vi "y1y2 副本.vi"(6 "二值化输入":u8[][](array[numeric]), 9 "Image Pixels (U8)输入":u8[][](array[numeric])) -> (0 "out right point 2":cluster{i32, i32}[](array[cluster]), 1 "right":cluster{i32, i32}[](graph), 2 "out left point":cluster{i32, i32}[](array[cluster]), 3 "left":cluster{i32, i32}[](graph), 4 "四个角点":i32[][](array[numeric]))   [LabVIEW 2014]
panel:
  out "x2max":cluster{i32, i32}
  out "x2min":cluster{i32, i32}
  out "x1min":cluster{i32, i32}
  out "x1max":cluster{i32, i32}
  # "x"
  # "1"
  # "2"
  # "y"
  # "x"
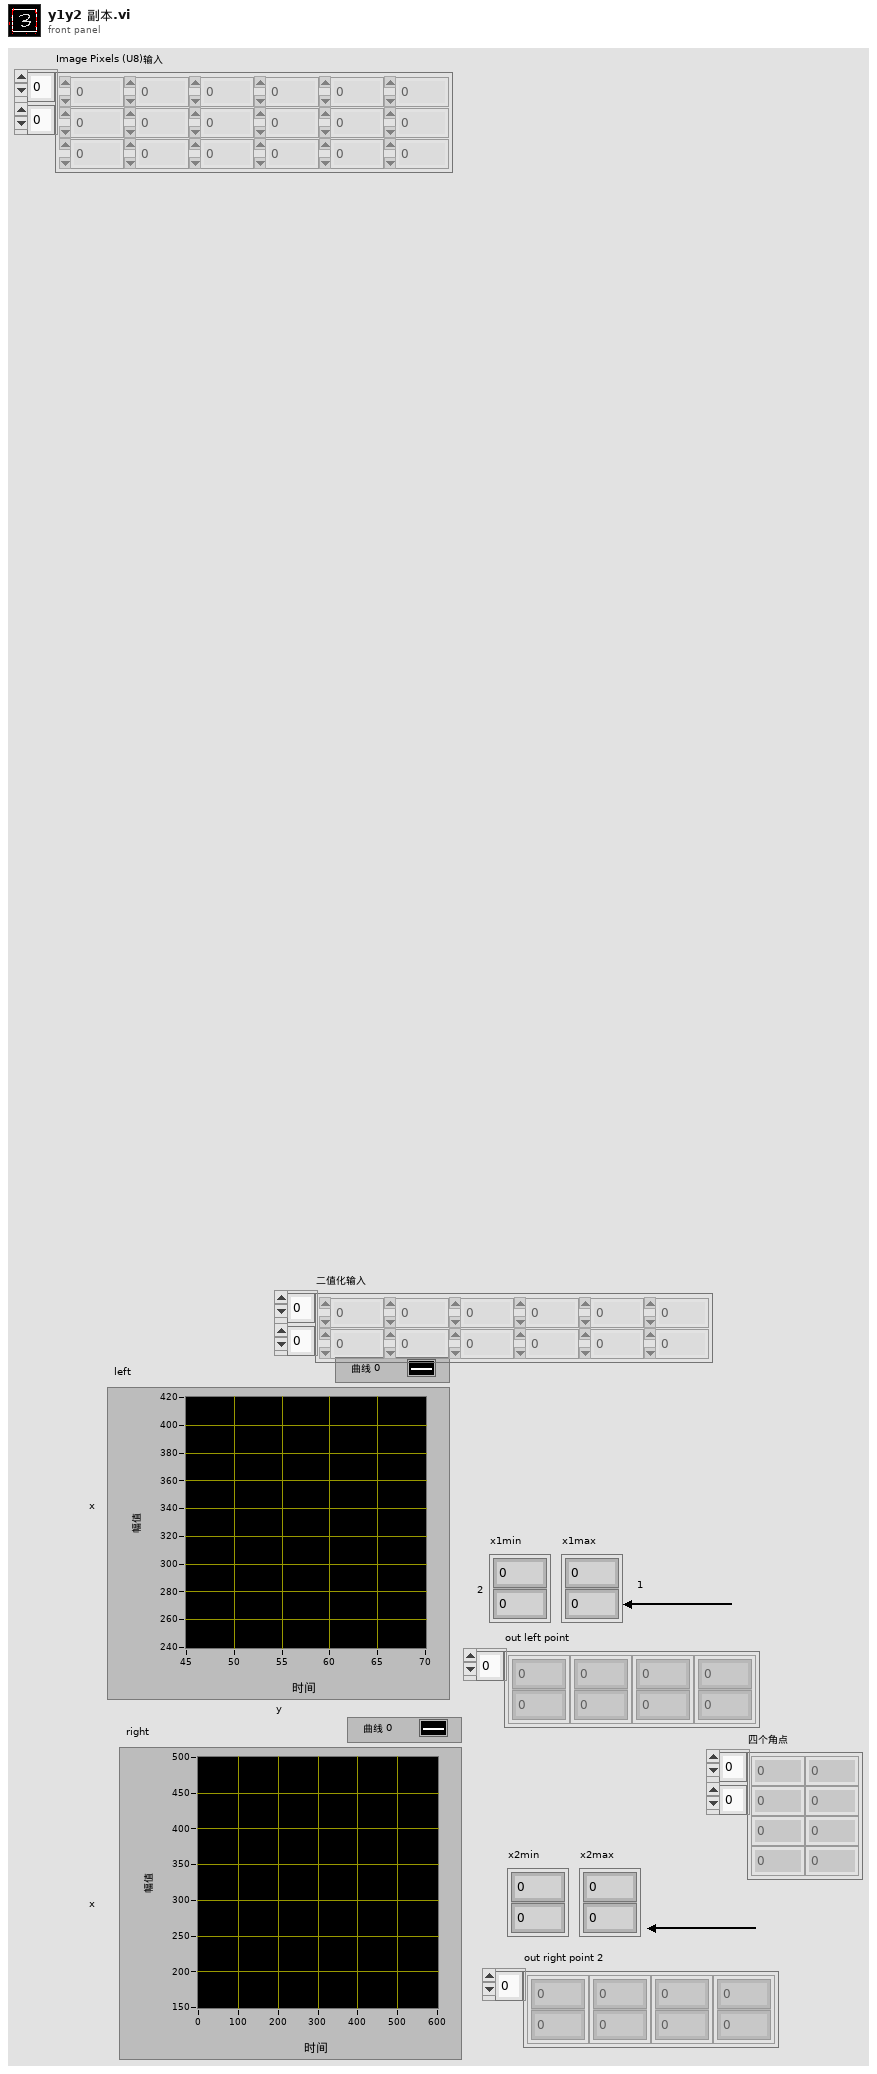
[diagram p1: front panel]
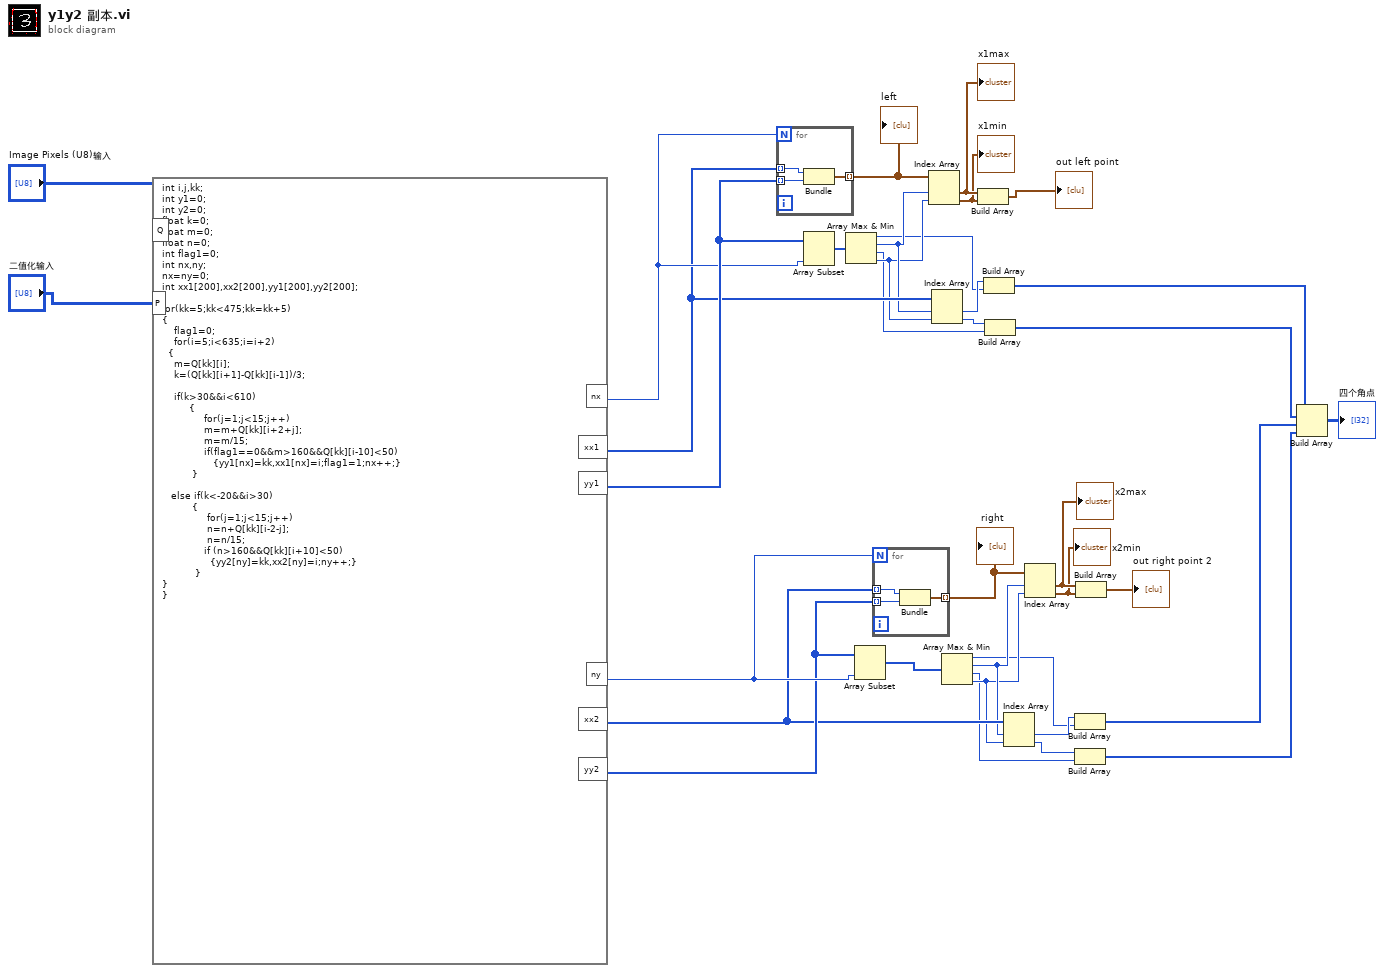
[diagram p0: block diagram]
diagram:
  n1 = formula code="int i,j,kk;\nint y1=0;\nint y2=0;\nfloat k=0;\nfloat m=0;\nfloat n=0;\nint flag1=0;\nint nx,ny;\nnx=ny=0;\nint xx1[200],xx2[200],yy1[200],yy2[200];\n\nfor(kk=5;kk<475;kk=kk+5)\n{\n    flag1=0;\n    for(i=5;i<635;i=i+2)\n  {\n    m=Q[kk][i];\n    k=(Q[kk][i+1]-Q[kk][i-1])/3;\n\n    if(k>30&&i<610)\n         {   \n              for(j=1;j<15;j++)\n              m=m+Q[kk][i+2+j];\n              m=m/15;\n              if(flag1==0&&m>160&&Q[kk][i-10]<50)\n                 {yy1[nx]=kk,xx1[nx]=i;flag1=1;nx++;}\n          }\n\n   else if(k<-20&&i>30)\n          {                   \n               for(j=1;j<15;j++)\n               n=n+Q[kk][i-2-j];\n               n=n/15;\n              if (n>160&&Q[kk][i+10]<50)\n                {yy2[ny]=kk,xx2[ny]=i;ny++;}\n           }\n}\n}"("Q"="Image Pixels (U8)输入", "P"="二值化输入") -> ("xx1"=w20:i32[], "yy1"=w34:i32[], "nx"=w33:i32, "xx2"=w10:i32[], "yy2"=w30:i32[], "ny"=w31:i32)
  n2 = for {
    N: w33 -> [_]
    tunnel: w20 -> [w38] mode=indexing
    tunnel: w34 -> [w37] mode=indexing
    tunnel: [w36] -> w35 mode=indexing
    n3 = Bundle(w38, w37) -> (w36:cluster{i32, i32})  [unwired: 1 in]
  }
  "left" <- w35
  n4 = Array Subset(array=w34, length=w33) -> (w23:i32[])  [unwired: 1 in]
  n5 = Array Max & Min(array=w23) -> (max value=w16:i32, max index (indices)=w19:i32, min value=w14:i32, min index (indices)=w18:i32)
  n6 = Array Subset(array=w30, length=w31) -> (w21:i32[])  [unwired: 1 in]
  n7 = for {
    N: w31 -> [_]
    tunnel: w10 -> [w41] mode=indexing
    tunnel: w30 -> [w40] mode=indexing
    tunnel: [w39] -> w32 mode=indexing
    n8 = Bundle(w41, w40) -> (w39:cluster{i32, i32})  [unwired: 1 in]
  }
  "right" <- w32
  n9 = Index Array(array=w35, index #1=w19, index #2=w18) -> (element #1=w28:cluster{i32, i32}, element #2=w27:cluster{i32, i32})
  "x1max" <- w28
  "x1min" <- w27
  n10 = Index Array(array=w20, index #1=w19, index #2=w18) -> (element #1=w17:i32, element #2=w15:i32)
  n11 = Array Max & Min(array=w21) -> (max value=w6:i32, max index (indices)=w8:i32, min value=w4:i32, min index (indices)=w7:i32)
  n12 = Build Array(w28, w27) -> (→"out left point":cluster{i32, i32}[])
  n13 = Build Array(w17, w16) -> (w13:i32[])
  n14 = Build Array(w15, w14) -> (w12:i32[])
  n15 = Index Array(array=w10, index #1=w8, index #2=w7) -> (element #1=w9:i32, element #2=w5:i32)
  n16 = Index Array(array=w32, index #1=w8, index #2=w7) -> (element #1=w25:cluster{i32, i32}, element #2=w24:cluster{i32, i32})
  "x2max" <- w25
  "x2min" <- w24
  n17 = Build Array(w9, w6) -> (w3:i32[])
  n18 = Build Array(w5, w4) -> (w2:i32[])
  n19 = Build Array(w25, w24) -> (→"out right point 2":cluster{i32, i32}[])
  n20 = Build Array(w13, w12, w3, w2) -> (→"四个角点":i32[][])
